vi "CS_cRIO-PB_MSAC2_DPV1-ReadWrite.vi"(0 "FPGA VI Reference":T1, 2 "DPV1-Service":i8(ring)=3 items=["Initiate", "Read", "Write", "Abort"], 5 "Slave":i8, 7 "Data":u8[](array[numeric]) format="%.0x", 11 "Error":errorcluster) -> (4 "FPGA VI Reference out":T1, 8 "Data out":u8[](array[numeric]) format="%.0x", 10 "Status":u8 format="%.0x", 15 "Error out":errorcluster)   [LabVIEW 2013, in "dynamic profibus.lvlib"]
doc: "Handles the cyclic process data of the selected DP-Slave.\n\nFPGA VI Reference:\nReference of the FPGA VI.\n\nSlave:\nPROFIBUS address of the DP-Slave. \n\nModify output data:\nThe Modify output data array contains the DP-Slave output data to be changed.\n\nInput data:\nThe Input data array contains the DP-Slave input data.\n\nOutput data:\nThe Output data array contains the DP-Slave output data.\n\nInput length:\nReturns the configured input length of the DP-Slave.\n\nOutput length:\nReturns the configured output length of the DP-Slave.\n\nSlave status:\n0x00: DP-Slave is in DataExchange mode, input and output data are valid\n0xC3: DP-Slave is not in Data Exchange mode, input and output data are invalid, DP-Slave diagnostic data are reported in Diag data array\n0xFF: DP-Slave is in Data Exchange mode and reports ext. diagnostic data, input and output data are valid.\n\nFPGA VI Reference out:\nIs a copy of the FPGA VI Reference .\n\nError in:\nPreceding error conditions. If an error has already occurred, the VI returns the value of the error in Error out.\n\nError out:\nError: TRUE if an error occurred.\nStatus: Error code\nInfo: Error description"
uses:
  dynamic profibus.lvlib
  CS_cRIO-PB_DP-Master_FPGA-Reference.ctl
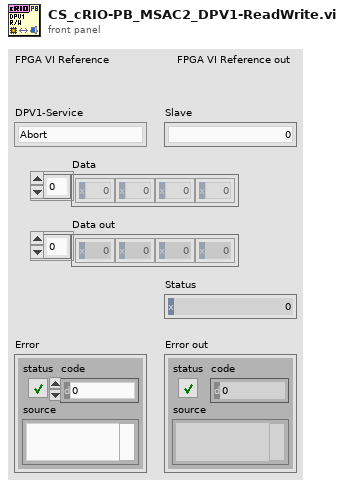
[diagram p1: front panel]
types:
  T1 = typedef "dynamic profibus.lvlib/CS_cRIO-PB_DP-Master_FPGA-Reference.ctl" = refnum<k20>
  T2 = enum16{"Start/Stop DP-Master", "Get Input Data", "Set Output Data", "Get Output Data", "Get Diagnostic Data", "Read/Write Data", "Read Diagnostic Data", "Get DPV1 Data", "Set DPV1 Data", "Read/Write DPV1 Data"}
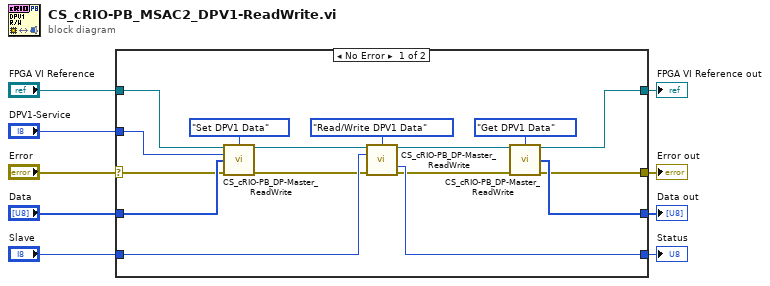
[diagram p0: block diagram]
diagram:
  n1 = case shown="No Error" "Error" {
    selector: "Error" -> [w19 w26]
    tunnel: "FPGA VI Reference" -> [w21 w27]
    tunnel: [w15 w27] -> w9
    tunnel: [w16 w26] -> w5
    tunnel: "Data" -> [w24 _]
    tunnel: "DPV1-Service" -> [w13 _]
    tunnel: "Slave" -> [w25 _]
    tunnel: [w23 _] -> w2
    tunnel: [w22 _] -> w1
    frame No Error {
      n2 = call "CS_cRIO-PB_DP-Master_ReadWrite.vi"("FPGA VI Reference"=w21, "Mode"=T2."Set DPV1 Data", "Slave"=w13, "Data"=w24, "Error"=w19) -> ("FPGA VI Reference out"=w14:T1, "Error out"=w20:errorcluster)  [unwired: 7 in, 2 out]
      n3 = call "CS_cRIO-PB_DP-Master_ReadWrite.vi"("FPGA VI Reference"=w14, "Mode"=T2."Read/Write DPV1 Data", "Slave"=w25, "Error"=w20) -> ("FPGA VI Reference out"=w18:T1, "Status"=w23:u8, "Error out"=w17:errorcluster)  [unwired: 8 in, 1 out]
      n4 = call "CS_cRIO-PB_DP-Master_ReadWrite.vi"("FPGA VI Reference"=w18, "Mode"=T2."Get DPV1 Data", "Error"=w17) -> ("FPGA VI Reference out"=w15:T1, "Data out"=w22:u8[], "Error out"=w16:errorcluster)  [unwired: 9 in, 1 out]
    }
    frame Error {
    }
  }
  "FPGA VI Reference out" <- w9
  "Error out" <- w5
  "Data out" <- w1
  "Status" <- w2
